vi "test_fecth_daq.vi"() -> ()   [LabVIEW 2014]
uses:
  common/crest/LabVIEW/LV14/libcommon-crest.lvlib
panel:
  out "tot of buf word":i32
  out "timestemp":string
  out "CU name":string
  out "data":string[](array[string])
  out "values out":string
  in  "!CHAOS WAN url":string="192.168.150.91:8081"
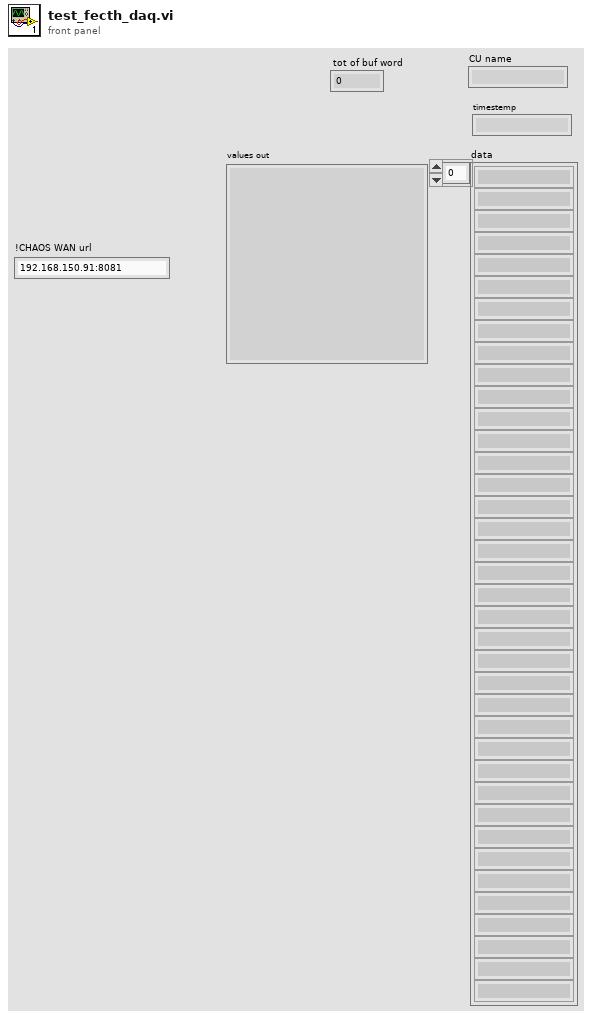
[diagram p1: front panel]
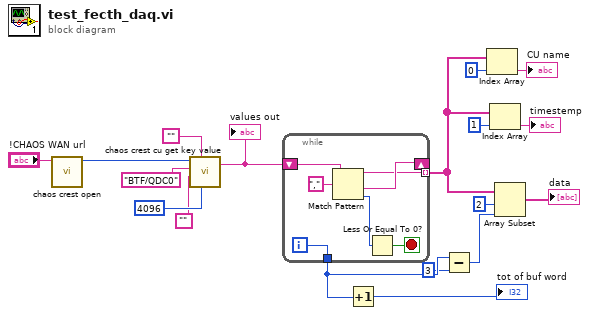
[diagram p0: block diagram]
diagram:
  n1 = call "chaos crest open.vi"("chaoswanurl"="!CHAOS WAN url") -> ("handleConnection"=w13:u32)  [unwired: 10 in]
  n2 = call "chaos crest cu get key value.vi"("maxsize"=4096, "values"="", "keys"="", "cuname"="BTF/QDC0", "handleConnection"=w13) -> ("values out"=w12:string)  [unwired: 3 in, 3 out]
  "values out" <- w12
  n3 = while {
    shift-right: [w23] -> _
    shift-left: w12 -> [w24]
    tunnel: [w22] -> w6 mode=indexing
    tunnel: [w19] -> w4
    i -> [w19]
    stop <- w21 stop-if-true
    n4 = Match Pattern(string=w24, regular expression=",") -> (before substring=w22:string, after substring=w23:string, offset past match=w20:i32)  [unwired: 1 in, 1 out]
    n5 = Less Or Equal To 0?(x=w20) -> (x <= 0?=w21:bool)
  }
  n6 = Increment(x=w4) -> (x+1=→"tot of buf word":i32)
  n7 = Subtract(x=w4, y=3) -> (x-y=w2:i32)
  n8 = Index Array(array=w6, index=0) -> (element=→"CU name":string)
  n9 = Index Array(array=w6, index=1) -> (element=→"timestemp":string)
  n10 = Array Subset(array=w6, index=2, length=w2) -> (→"data":string[])
